vi "Convert_Meters_to_Inches_Array.vi"(4 "Meters":dbl[](array[numeric])) -> (1 "Inches":dbl[](array[numeric]))   [LabVIEW 2011]
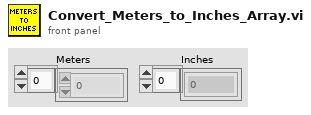
[diagram p1: front panel]
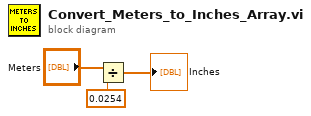
[diagram p0: block diagram]
diagram:
  n1 = Divide(x="Meters", y=0.0254) -> (x/y=→"Inches":dbl[])
